vi "Read Set.vi"(0 "VISA resource name":refnum<visa-resource-name>, 11 "error in (no error)":errorcluster) -> (1 "Local Lockout":u32(ring) items=["Off", "On"], 2 "ATTN":u32(ring) items=["Off", "On"], 3 "Run/Stop":u32(ring)=1 items=["Stop", "Run"], 4 "VISA resource name out":refnum<visa-resource-name>, 5 "Wavelength (nnnn)":dbl[unit], 6 "AVG":u32(ring) items=["Slow", "Medium", "Fast"], 9 "Range (1:8)":u32(ring) items=["Auto", "Lowest", "2", "3", "4", "5", "6", "7", "Highest"], 10 "Units":u32(ring)=1 items=["W"=1, "dB"=2, "dBm"=3, "REL"=4], 12 "Backlight":u32(ring) items=["Off", "Low", "High"], 13 "Beeper":u32(ring) items=["Off", "On"], 14 "Zero":u32(ring) items=["Off", "On"], 15 "error out":errorcluster)   [LabVIEW 2009]
doc: "Reads 1830-C options in succession and outputs their values.\n\nNote: Cannot tell if AutoRange is active."
uses:
  Newport 1830-C/Newport 1830-C.lvlib
panel:
  in  "milliseconds to wait":u32=100
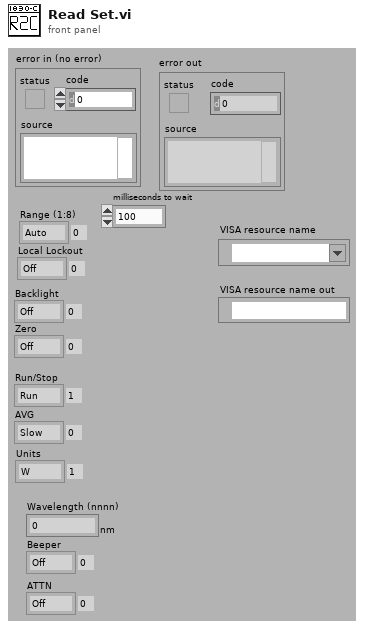
[diagram p1: front panel]
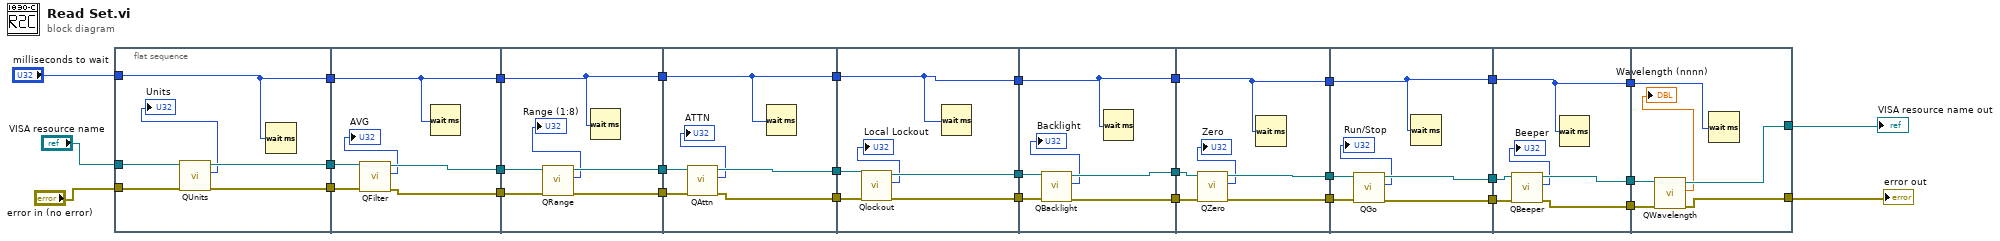
[diagram p0: block diagram]
diagram:
  n1 = flat-sequence {
    tunnel: [w38] -> w32
    tunnel: [w35] -> w22
    tunnel: "milliseconds to wait" -> [w35]
    tunnel: "VISA resource name" -> [w37]
    tunnel: "error in (no error)" -> [w36]
    tunnel: [w34] -> w10
    tunnel: w32 -> [w44]
    tunnel: [w43] -> w31
    tunnel: w22 -> [w42]
    tunnel: [w42] -> w21
    tunnel: w10 -> [w41]
    tunnel: [w40] -> w9
    tunnel: w31 -> [w50]
    tunnel: [w49] -> w30
    tunnel: w21 -> [w48]
    tunnel: [w48] -> w20
    tunnel: w9 -> [w47]
    tunnel: [w46] -> w8
    tunnel: w30 -> [w56]
    tunnel: [w55] -> w29
    tunnel: w20 -> [w54]
    tunnel: [w54] -> w19
    tunnel: w8 -> [w53]
    tunnel: [w52] -> w7
    tunnel: w29 -> [w62]
    tunnel: [w61] -> w28
    tunnel: w19 -> [w60]
    tunnel: [w60] -> w18
    tunnel: w7 -> [w59]
    tunnel: [w58] -> w6
    tunnel: w28 -> [w68]
    tunnel: [w67] -> w27
    tunnel: w18 -> [w66]
    tunnel: [w66] -> w17
    tunnel: w6 -> [w65]
    tunnel: [w64] -> w5
    tunnel: w27 -> [w74]
    tunnel: [w73] -> w26
    tunnel: w17 -> [w72]
    tunnel: [w72] -> w16
    tunnel: w5 -> [w71]
    tunnel: [w70] -> w4
    tunnel: w26 -> [w80]
    tunnel: [w79] -> w25
    tunnel: w16 -> [w78]
    tunnel: [w78] -> w15
    tunnel: w4 -> [w77]
    tunnel: [w76] -> w3
    tunnel: w25 -> [w86]
    tunnel: [w85] -> w24
    tunnel: w15 -> [w84]
    tunnel: [w84] -> w14
    tunnel: w3 -> [w83]
    tunnel: [w82] -> w2
    tunnel: w24 -> [w92]
    tunnel: [w91] -> w23
    tunnel: w14 -> [w90]
    tunnel: w2 -> [w89]
    tunnel: [w88] -> w1
    frame #0 {
      n2 = call "QUnits.vi"("error in (no error)"=w36, "VISA resource name"=w37) -> ("error out"=w34:errorcluster, "Units"=→"Units":u32, "VISA resource name out"=w38:refnum<visa-resource-name>)  [unwired: 6 in, 1 out]
      n3 = Wait (ms)(milliseconds to wait=w35) -> ()  [unwired: 1 out]
    }
    frame #1 {
      n4 = call "QFilter.vi"("error in (no error)"=w41, "VISA resource name"=w44) -> ("error out"=w40:errorcluster, "Filter State"=→"AVG":u32, "VISA resource name out"=w43:refnum<visa-resource-name>)  [unwired: 7 in]
      n5 = Wait (ms)(milliseconds to wait=w42) -> ()  [unwired: 1 out]
    }
    frame #2 {
      n6 = call "QRange.vi"("error in (no error)"=w47, "VISA resource name"=w50) -> ("error out"=w46:errorcluster, "Range"=→"Range (1:8)":u32, "VISA resource name out"=w49:refnum<visa-resource-name>)  [unwired: 7 in]
      n7 = Wait (ms)(milliseconds to wait=w48) -> ()  [unwired: 1 out]
    }
    frame #3 {
      n8 = call "QAttn.vi"("error in (no error)"=w53, "VISA resource name"=w56) -> ("error out"=w52:errorcluster, "Attn State"=→"ATTN":u32, "VISA resource name out"=w55:refnum<visa-resource-name>)  [unwired: 7 in]
      n9 = Wait (ms)(milliseconds to wait=w54) -> ()  [unwired: 1 out]
    }
    frame #4 {
      n10 = call "Qlockout.vi"("error in (no error)"=w59, "VISA resource name"=w62) -> ("error out"=w58:errorcluster, "Lockout State"=→"Local Lockout":u32, "VISA resource name out"=w61:refnum<visa-resource-name>)  [unwired: 7 in]
      n11 = Wait (ms)(milliseconds to wait=w60) -> ()  [unwired: 1 out]
    }
    frame #5 {
      n12 = call "QBacklight.vi"("error in (no error)"=w65, "VISA resource name"=w68) -> ("error out"=w64:errorcluster, "BKLT State"=→"Backlight":u32, "VISA resource name out"=w67:refnum<visa-resource-name>)  [unwired: 7 in]
      n13 = Wait (ms)(milliseconds to wait=w66) -> ()  [unwired: 1 out]
    }
    frame #6 {
      n14 = call "QZero.vi"("error in (no error)"=w71, "VISA resource name"=w74) -> ("error out"=w70:errorcluster, "Zero State"=→"Zero":u32, "VISA resource name out"=w73:refnum<visa-resource-name>)  [unwired: 7 in]
      n15 = Wait (ms)(milliseconds to wait=w72) -> ()  [unwired: 1 out]
    }
    frame #7 {
      n16 = call "QGo.vi"("error in (no error)"=w77, "VISA resource name"=w80) -> ("error out"=w76:errorcluster, "Go State"=→"Run/Stop":u32, "VISA resource name out"=w79:refnum<visa-resource-name>)  [unwired: 7 in]
      n17 = Wait (ms)(milliseconds to wait=w78) -> ()  [unwired: 1 out]
    }
    frame #8 {
      n18 = call "QBeeper.vi"("error in (no error)"=w83, "VISA resource name"=w86) -> ("error out"=w82:errorcluster, "Beeper State"=→"Beeper":u32, "VISA resource name out"=w85:refnum<visa-resource-name>)  [unwired: 7 in]
      n19 = Wait (ms)(milliseconds to wait=w84) -> ()  [unwired: 1 out]
    }
    frame #9 {
      n20 = call "QWavelength.vi"("error in (no error)"=w89, "VISA resource name"=w92) -> ("error out"=w88:errorcluster, "Wavelength"=→"Wavelength (nnnn)":dbl[unit], "VISA resource name out"=w91:refnum<visa-resource-name>)  [unwired: 7 in]
      n21 = Wait (ms)(milliseconds to wait=w90) -> ()  [unwired: 1 out]
    }
  }
  "error out" <- w1
  "VISA resource name out" <- w23
